vi "FindMinimumChiSquared.vi"(0 "X Mean std error Expected extinction":T2, 1 "max size parameter alpha\n(alpha = 2Pi*r/lambda)":sgl=1.0 step=0.01 format="%.2f") -> (2 "Chi Squared Surface":dbl[][](array[numeric]), 3 "Real Part from fit":dbl=1.3, 4 "Imaginary Part from fit":dbl=0.1)   [LabVIEW 2011]
uses:
  <vilib>/Math Plots/3D Math Plots/3D Contour/3D Contour XCtrl/3D Contour.xctl
  <vilib>/Math Plots/3D Math Plots/3D Contour/3D Contour Datatype/3D Contour Datatype.lvclass
  <vilib>/Analysis/1siggen.llb/Ramp Pattern by Samples.vi
  <vilib>/Math Plots/3D Math Plots/3D Contour/3D Contour Datatype/Public/Plot Helper (Matrix).vi
  Software/Labview optimization vi/RTDownhillSimplex.llb/RTDownhillSimplexGlobals.vi
  <vilib>/Analysis/NI_AALBase.lvlib
panel:
  out "Stopping condition flag":bool
  out "x-y":dbl[](array[numeric])
  in  "buzzer":bool
  in  "Continous":bool=TRUE
  in  "sleep-time":dbl
  out "Simplex":cluster{dbl[], dbl[]}(graph)={[0.9999999941783686, 1.0000000000877893, 0.9999999991380464, 0.9999999941783686], [0.9999999882799789, 0.9999999995794436, 0.9999999977588435, 0.9999999882799789]}
  out "ValueInput":dbl
  out "ValueOutput":dbl
  out "newSimplexPoint":dbl[](array[numeric])
  in  "Testfunction":enum16{"Rosenbrock function", "PID Controller"}(ring)=enum."PID Controller"
  out "level curves":dbl[][](graph)
  in  "Starting points":dbl[][](array[numeric])=[[0.8, 1.7, 1.7], [0.85, 1.7, 1.7], [0.8, 1.75, 1.7], [0.8, 1.7, 1.75]]
  in  "Downhill-Simplex parameters":T1={"alpha"=1.0, "beta"=0.5, "gamma"=2.0, "Maximum"=TRUE}
  in  "Starting points 2":dbl[][](array[numeric])=[[1.7, 1.7], [1.75, 1.7], [1.7, 1.75]]
  out "min index(es)":i32[](array[numeric])=[0, 10]
  out "3D Contour":refnum<class "3D Plot Datatype.lvclass">[](xcontrol)
  out "Inside loop":i32=30
  out "Outside loop":i32=40
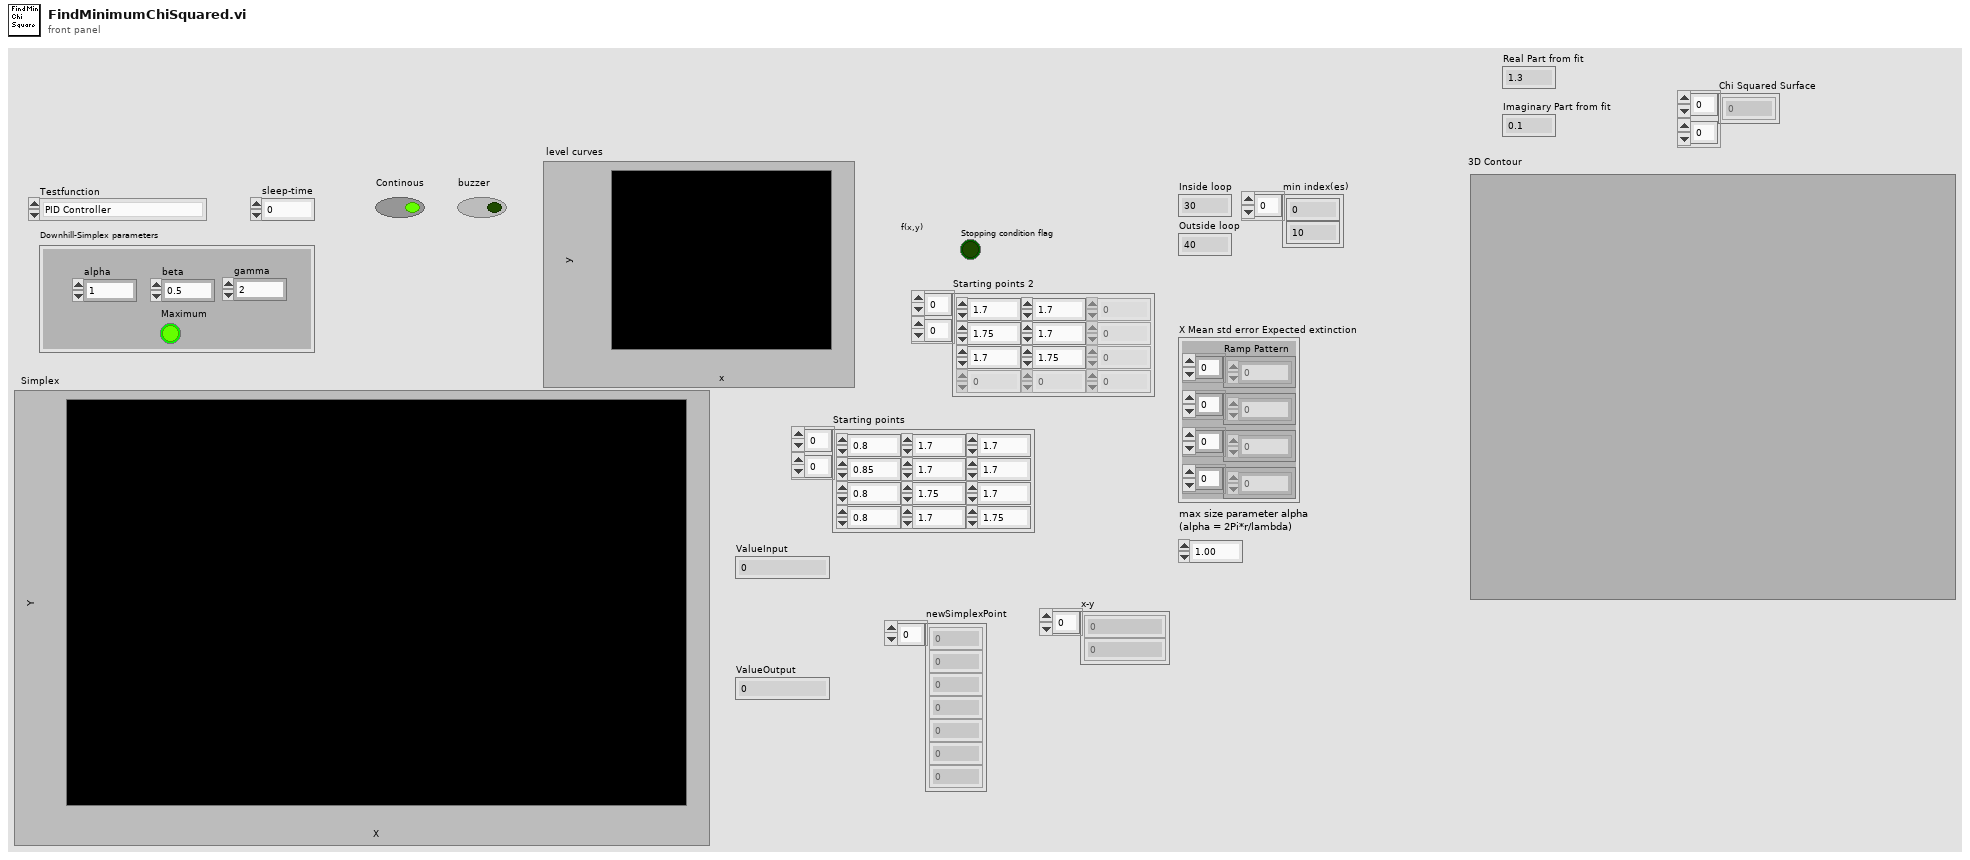
[diagram p1: front panel]
types:
  T1 = cluster{"alpha":dbl, "beta":dbl, "gamma":dbl, "Maximum":bool}
  T2 = cluster{"Ramp Pattern":dbl[], dbl[], dbl[], sgl[]}
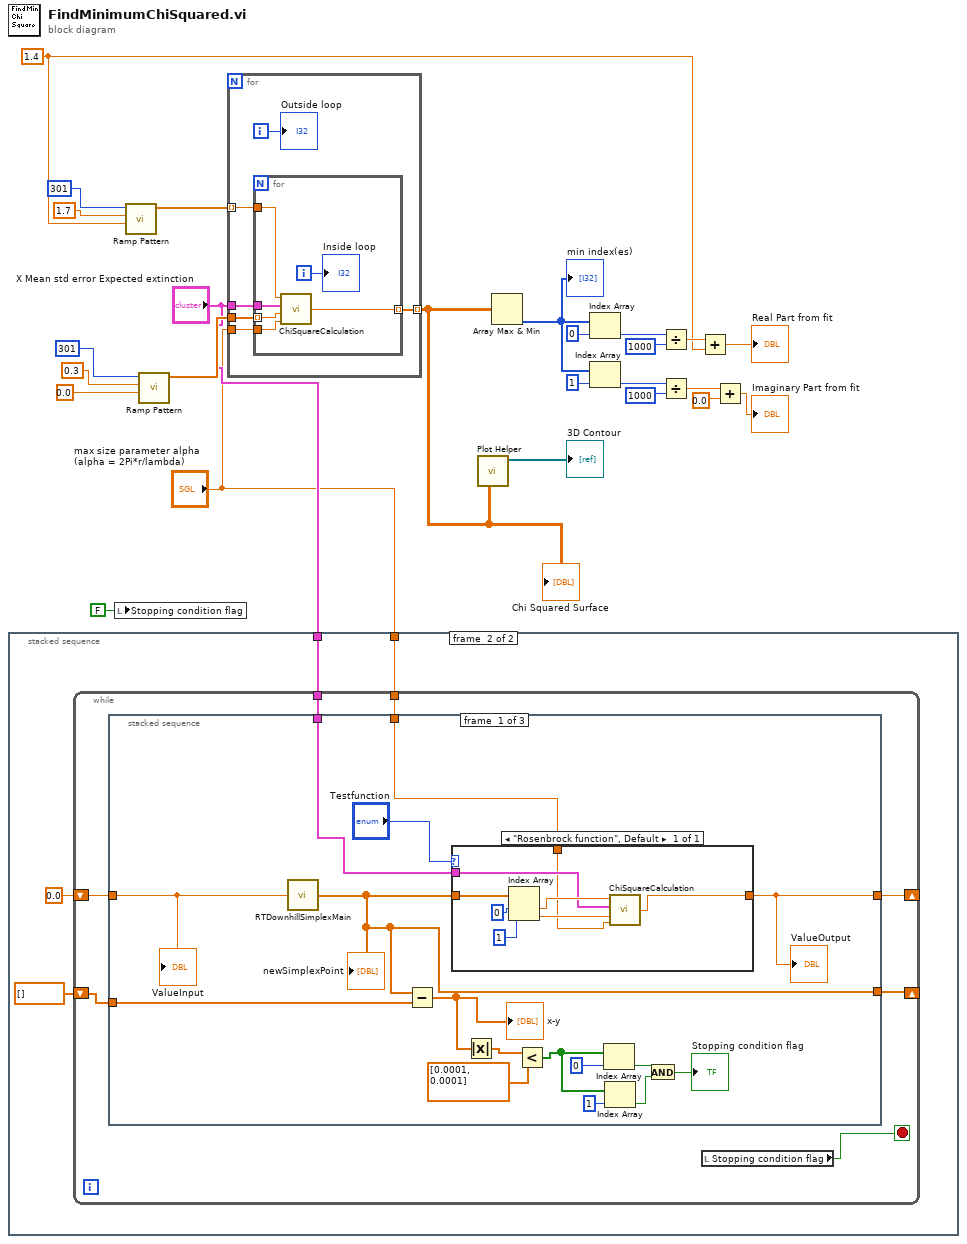
[diagram p0: block diagram]
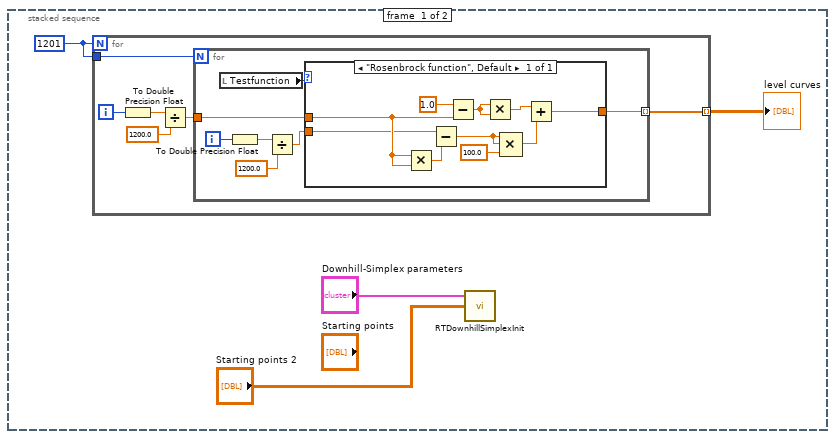
[diagram p2: hidden frame]
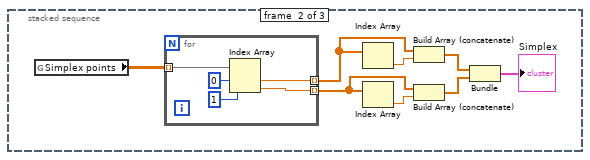
[diagram p3: hidden frame]
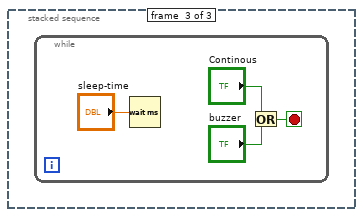
[diagram p4: hidden frame]
diagram:
  w6 = 1.4 ("start")
  n1 = stacked-sequence {
    tunnel: "X Mean std error Expected extinction" -> [_ w55]
    tunnel: "max size parameter alpha\n(alpha = 2Pi*r/lambda)" -> [_ w54]
    frame #0 {
      w28 = 1201
      n2 = for {
        N: w28 -> [_]
        tunnel: w28 -> [w31]
        tunnel: [w30] -> w27 mode=indexing
        i -> [w35]
        n3 = To Double Precision Float(number=w35) -> (double precision float=w34:dbl)
        n4 = Divide(x=w34, y=1200.0) -> (x/y=w32:dbl)
        n5 = for {
          N: w31 -> [_]
          tunnel: w32 -> [w39]
          tunnel: [w37] -> w30 mode=indexing
          i -> [w40]
          n6 = local read "Testfunction"() -> (w36:enum16{"Rosenbrock function", "PID Controller"})
          n7 = To Double Precision Float(number=w40) -> (double precision float=w41:dbl)
          n8 = Divide(x=w41, y=1200.0) -> (x/y=w38:dbl)
          n9 = case shown="\"Rosenbrock function\", Default" w36 {
            tunnel: [w45] -> w37
            tunnel: w39 -> [w44]
            tunnel: w38 -> [w43]
            frame "Rosenbrock function", Default {
              n10 = Multiply(x=w44, y=w44) -> (x*y=w48:dbl)
              n11 = Subtract(x=w43, y=w48) -> (x-y=w47:dbl)
              n12 = Subtract(x=1.0, y=w44) -> (x-y=w51:dbl)
              n13 = Multiply(x=w51, y=w51) -> (x*y=w50:dbl)
              n14 = Compound Arithmetic op=MULTIPLY(w47, w47, 100.0 ("value")) -> (w46:dbl)
              n15 = Add(x=w50, y=w46) -> (x+y=w45:dbl)
            }
          }
        }
      }
      "level curves" <- w27
      n16 = call "RTDownhillSimplexInit.vi"("Starting points"="Starting points 2", "Downhill-Simplex parameters"="Downhill-Simplex parameters") -> ()  [unwired: 2 in]
    }
    frame #1 {
      n17 = while {
        shift-right: [w60] -> _
        shift-left: 0.0 -> [w63]
        tunnel: w55 -> [w62]
        tunnel: w54 -> [w61]
        shift-right: [w59] -> _
        shift-left: dbl[] [] ("newSimplexPoint") -> [w58]
        stop <- w57 stop-if-true
        n18 = stacked-sequence {
          tunnel: w63 -> [w79 _ _]
          tunnel: w62 -> [w77 _ _]
          tunnel: w61 -> [w76 _ _]
          tunnel: [w75 _ _] -> w60
          tunnel: [w74 _ _] -> w59
          tunnel: w58 -> [w73 _ _]
          frame #0 {
            n19 = call "RTDownhillSimplexMain.vi"("newSimplexValue"=w79) -> ("newSimplexPoint"=w74:dbl[])
            "newSimplexPoint" <- w74
            n20 = Subtract(x=w74, y=w73) -> (x-y=w72:dbl[])
            "x-y" <- w72
            n21 = case shown="\"Rosenbrock function\", Default" "Testfunction" {
              tunnel: w74 -> [w87]
              tunnel: w77 -> [w82]
              tunnel: w76 -> [w81]
              tunnel: [w80] -> w75
              frame "Rosenbrock function", Default {
                n22 = Index Array(array=w87, index #1=0 ("index"), index #2=1 ("index")) -> (element #1=w84:dbl, element #2=w83:dbl)
                n23 = call "ChiSquareCalculation.vi"("max size parameter alpha\n(alpha = 2Pi*r/lambda)"=w81, "refractive index, imaginary"=w83, "X Mean std error Expected extinction"=w82, "refractive index, real"=w84) -> ("Chi Squared"=w80:dbl)
              }
            }
            "ValueOutput" <- w75
            n24 = Absolute Value(x=w72) -> (abs(x)=w71:dbl[])
            n25 = Less?(x=w71, y=dbl[] [0.0001, 0.0001]) -> (x < y?=w67:bool[])
            n26 = Index Array(array=w67, index=0) -> (element=w66:bool)
            n27 = Index Array(array=w67, index=1) -> (element=w65:bool)
            n28 = And(x=w66, y=w65) -> (x .and. y?=→"Stopping condition flag":bool)
            "ValueInput" <- w79
          }
          frame #1 {
            n29 = global read "RTDownhillSimplexGlobals.vi" "Simplex points"() -> (w88:dbl[][])
            n30 = for {
              tunnel: w88 -> [w100] mode=indexing
              tunnel: [w97] -> w94 mode=indexing
              tunnel: [w96] -> w91 mode=indexing
              n31 = Index Array(array=w100, index #1=0 ("index"), index #2=1 ("index")) -> (element #1=w97:dbl, element #2=w96:dbl)
            }
            n32 = Index Array(array=w94) -> (element=w95:dbl)  [unwired: 1 in]
            n33 = Index Array(array=w91) -> (element=w92:dbl)  [unwired: 1 in]
            n34 = Build Array (concatenate)(w94, w95) -> (w93:dbl[])
            n35 = Build Array (concatenate)(w91, w92) -> (w90:dbl[])
            n36 = Bundle(w93, w90) -> (→"Simplex":cluster{dbl[], dbl[]})  [unwired: 1 out]
          }
          frame #2 {
            n37 = while {
              stop <- w103 stop-if-true
              n38 = Wait (ms)(milliseconds to wait="sleep-time") -> ()  [unwired: 1 out]
              n39 = Or(x="Continous", y="buzzer") -> (x .or. y?=w103:bool)
            }
          }
        }
        n40 = local read "Stopping condition flag"() -> (w57:bool)
      }
    }
  }
  n41 = local write "Stopping condition flag"(FALSE ("Stopping condition flag")) -> ()
  n42 = call-poly <vilib>:"Ramp Pattern.vi"("start"=w6, "end"=1.7, "samples"=301) -> ("Ramp Pattern"=w20:dbl[])  [unwired: 7 in, 1 out]
  n43 = call-poly <vilib>:"Ramp Pattern.vi"("start"=0.0, "end"=0.3, "samples"=301) -> ("Ramp Pattern"=w19:dbl[])  [unwired: 7 in, 1 out]
  n44 = for {
    tunnel: w20 -> [w110] mode=indexing
    tunnel: w19 -> [w109]
    tunnel: [w108] -> w17 mode=indexing
    tunnel: "X Mean std error Expected extinction" -> [w106]
    tunnel: "max size parameter alpha\n(alpha = 2Pi*r/lambda)" -> [w105]
    i -> [w107]
    n45 = for {
      tunnel: w110 -> [w116]
      tunnel: w109 -> [w115] mode=indexing
      tunnel: [w114] -> w108 mode=indexing
      tunnel: w106 -> [w112]
      tunnel: w105 -> [w111]
      i -> [w113]
      n46 = call "ChiSquareCalculation.vi"("max size parameter alpha\n(alpha = 2Pi*r/lambda)"=w111, "refractive index, imaginary"=w115, "X Mean std error Expected extinction"=w112, "refractive index, real"=w116) -> ("Chi Squared"=w114:dbl)
      "Inside loop" <- w113
    }
    "Outside loop" <- w107
  }
  "Chi Squared Surface" <- w17
  n47 = call-poly <vilib>:"Plot Helper.vi"("z matrix"=w17) -> ("3D Plot lvclass Array out"=→"3D Contour":refnum<class "3D Plot Datatype.lvclass">[])  [unwired: 5 in, 5 out]
  n48 = Array Max & Min(array=w17) -> (min index (indices)=w14:i32[])  [unwired: 3 out]
  "min index(es)" <- w14
  n49 = Index Array(array=w14, index=0) -> (element=w13:i32)
  n50 = Index Array(array=w14, index=1) -> (element=w10:i32)
  n51 = Divide(x=w13, y=1000) -> (x/y=w8:dbl)
  n52 = Divide(x=w10, y=1000) -> (x/y=w9:dbl)
  n53 = Add(x=w8, y=w6) -> (x+y=→"Real Part from fit":dbl)
  n54 = Add(x=w9, y=0.0) -> (x+y=→"Imaginary Part from fit":dbl)
